vi "Convert NT Boolean to LV String.vi"(11 "Boolean":bool) -> (3 "string":string)   [LabVIEW 2017]
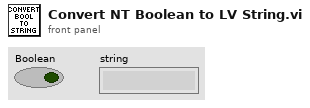
[diagram p1: front panel]
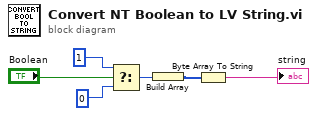
[diagram p0: block diagram]
diagram:
  n1 = Select(t=u8 1, s="Boolean", f=u8 0) -> (s? t:f=w5:u8)
  n2 = Build Array(w5) -> (w1:u8[])
  n3 = Byte Array To String(unsigned byte array=w1) -> (string=→"string":string)
